vi "reset FPGA DMA.vi"(2 "error in":errorcluster, 3 "FPGA VI Reference In":T1) -> (0 "error out":errorcluster, 1 "FPGA VI Reference Out":T1)   [LabVIEW 2014]
uses:
  openfpgaref.8.6.ctl
  <vilib>/Utility/error.llb/Error Cluster From Error Code.vi
  <vilib>/rvi/errors/niLvFpgaAdjustHostInterfaceError.vi
  <vilib>/rvi/interface/nirviReadWriteControl/nirviReadWriteControl.xnode
  FPGA Bitfiles/UHR-FleezersInst_FPGATarget_UHR-FleezersCont_avogadro5_symmetric.lvbitx
  <vilib>/rvi/interface/nirviMethod/nirviMethod.xnode
  <vilib>/rvi/errors/niLvFpgaMergeErrorWithErrorCode.vi
  <vilib>/FPGAPlugInAG/PCIe-7852R/niLvFpga_StopFifo_PCIe-7852R.vi
  <vilib>/FPGAPlugInAG/PCIe-7852R/niLvFpga_StartFifo_PCIe-7852R.vi
  NiFpgaLv.dll
panel:
  out "Overflow (data lost)":bool
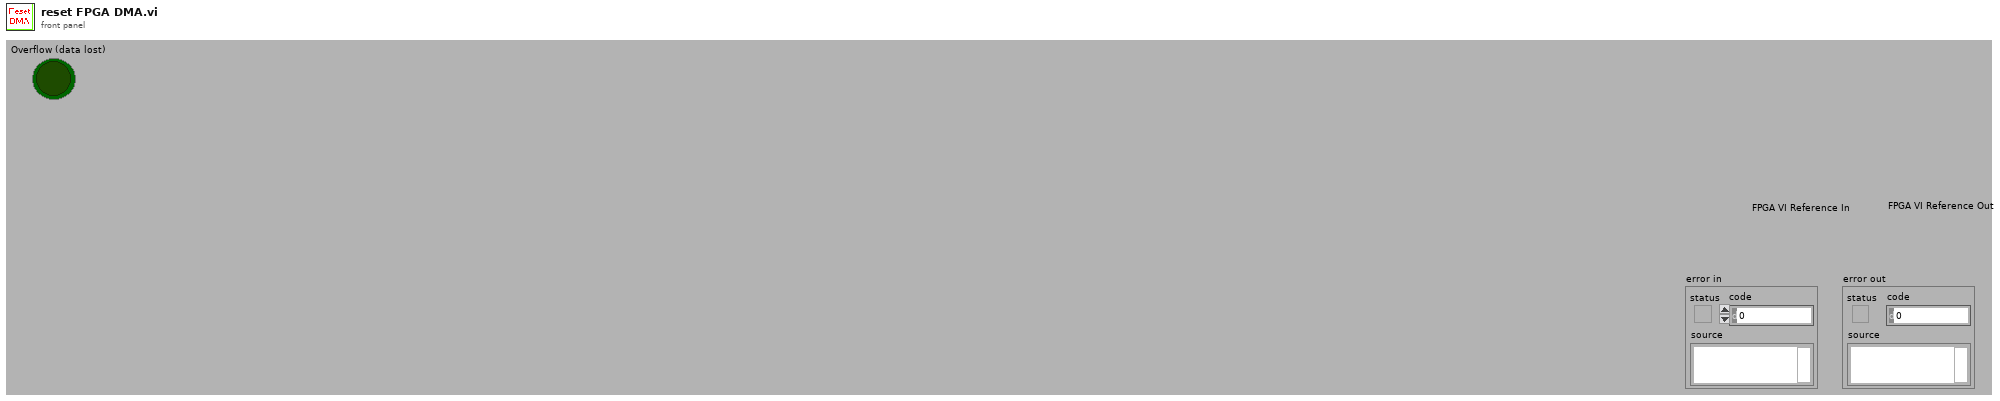
[diagram p1: front panel]
types:
  T1 = typedef "openfpgaref.8.6.ctl" = refnum<k20>
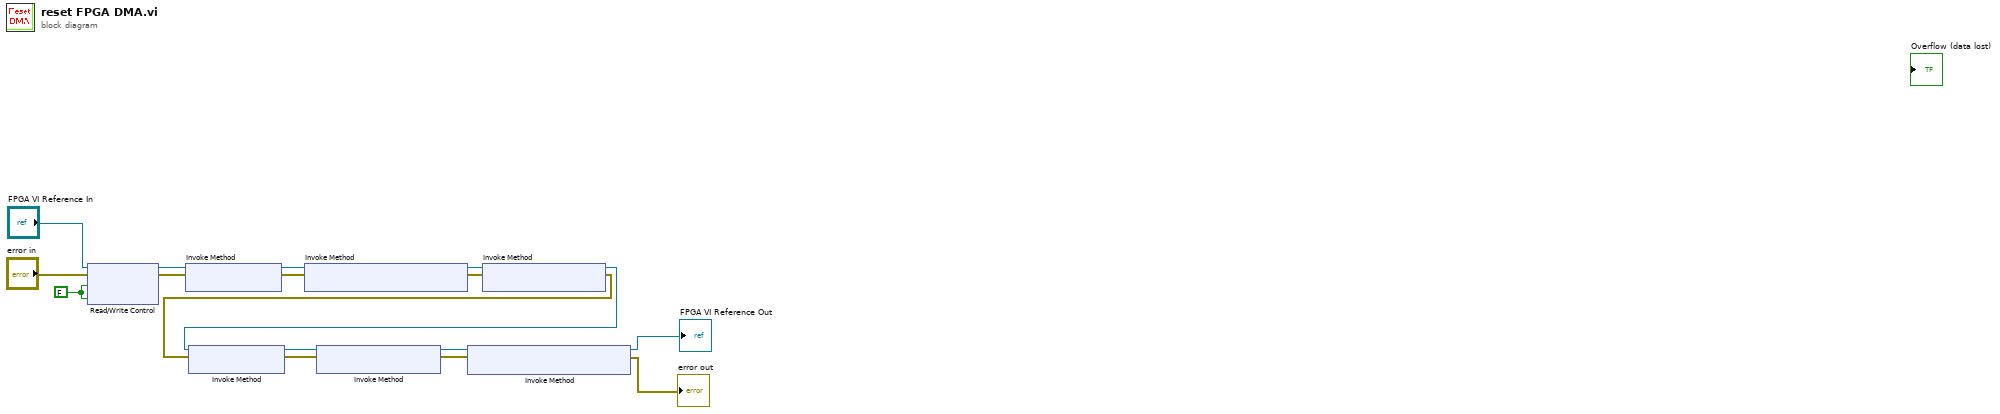
[diagram p0: block diagram]
diagram:
  w17 = FALSE ("AI to FIFO")
  n1 = xnode "Read/Write Control"("FPGA VI Reference In"="FPGA VI Reference In", "error in"="error in", "AI to FIFO"=w17, "APD to FIFO"=w17) -> ("FPGA VI Reference Out"=w6:T1, "error out"=w16:errorcluster)
  n2 = xnode "Invoke Method"("FPGA VI Reference In"=w6, "error in"=w16) -> ("FPGA VI Reference Out"=w14:T1, "error out"=w15:errorcluster)
  n3 = xnode "Invoke Method"("FPGA VI Reference In"=w14, "error in"=w15) -> ("FPGA VI Reference Out"=w13:T1, "error out"=w12:errorcluster)
  n4 = xnode "Invoke Method"("FPGA VI Reference In"=w13, "error in"=w12) -> ("FPGA VI Reference Out"=w11:T1, "error out"=w5:errorcluster)
  n5 = xnode "Invoke Method"("FPGA VI Reference In"=w11, "error in"=w5) -> ("FPGA VI Reference Out"=w10:T1, "error out"=w4:errorcluster)
  n6 = xnode "Invoke Method"("FPGA VI Reference In"=w10, "error in"=w4) -> ("FPGA VI Reference Out"=w9:T1, "error out"=w3:errorcluster)
  n7 = xnode "Invoke Method"("FPGA VI Reference In"=w9, "error in"=w3) -> ("FPGA VI Reference Out"=→"FPGA VI Reference Out":T1, "error out"=→"error out":errorcluster)
